vi "Edit_String_Options_list.vi"(2 "Channel Name":string, 3 "String array":string[](array[string])) -> (0 "New Selection Index":i32, 1 "String array Out":string[](array[string]))   [LabVIEW 2010]
uses:
  Controls/ok_button.ctl
panel:
  in  "Menu Strings":string[][](table)
  out "Meassage":string
  in  "OK":T1
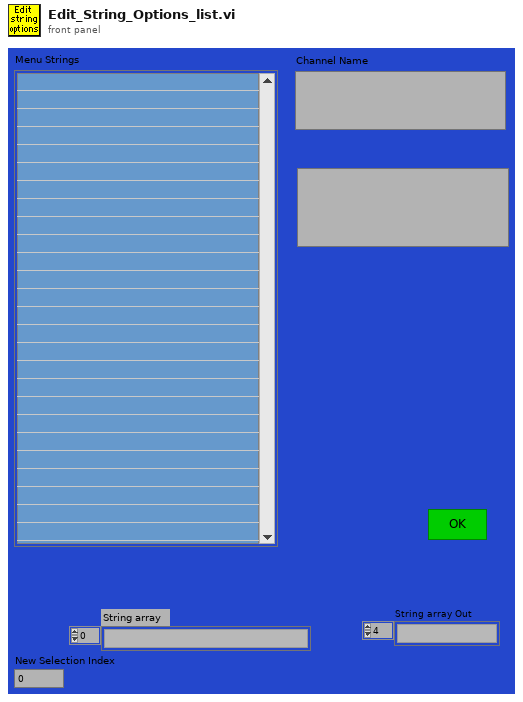
[diagram p1: front panel]
types:
  T1 = typedef "ok_button.ctl" = bool
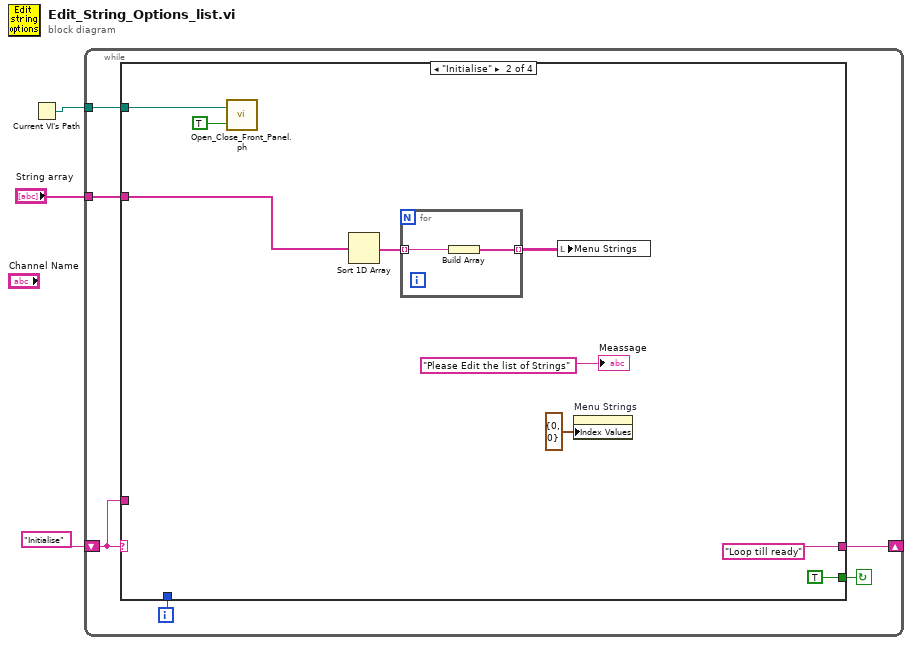
[diagram p0: block diagram]
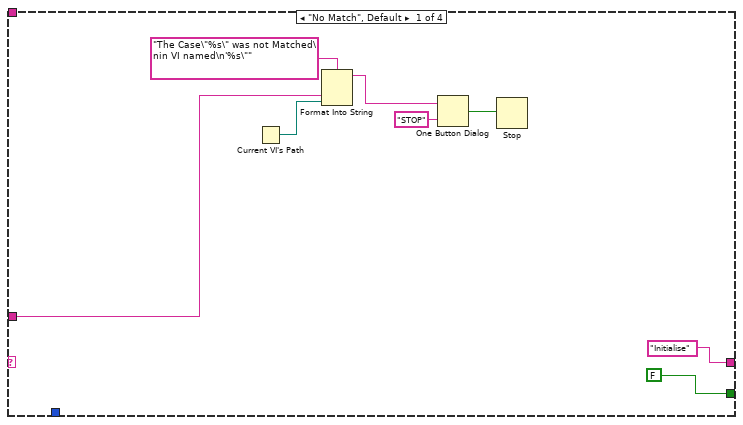
[diagram p2: hidden frame]
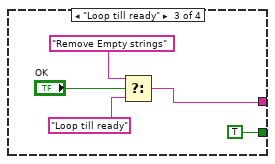
[diagram p3: hidden frame]
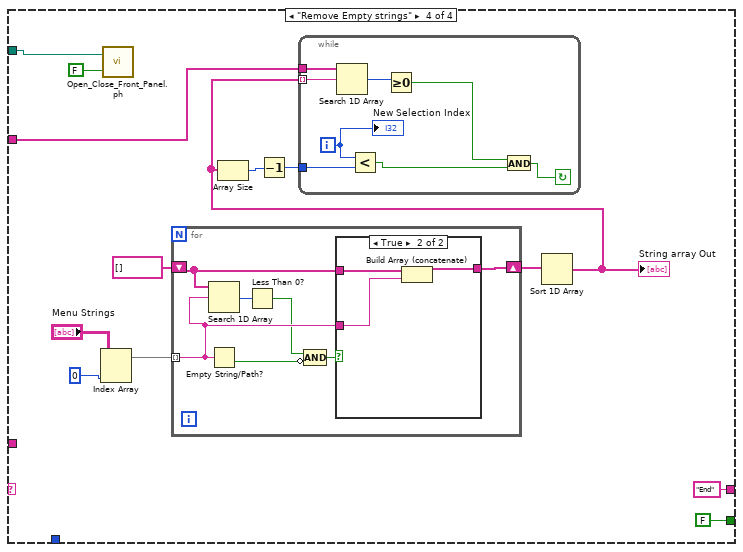
[diagram p4: hidden frame]
diagram:
  n1 = Current VI's Path() -> (path=w2:path)
  n2 = while {
    shift-left: "Initialise" -> [w7]
    shift-right: [w8] -> _
    tunnel: w2 -> [w5]
    tunnel: "String array" -> [w4]
    i -> [w6]
    stop <- w9 continue-if-true
    n3 = case shown="\"Initialise\"" w7 {
      tunnel: [FALSE TRUE TRUE FALSE] -> w9
      tunnel: ["Initialise" "Loop till ready" w30 "End"] -> w8
      tunnel: w7 -> [w12 _ _ _]
      tunnel: w6 -> [_ _ _ _]
      tunnel: w5 -> [_ w20 _ w38]
      tunnel: w4 -> [_ w18 _ w37]
      frame "No Match", Default {
        n4 = Current VI's Path() -> (path=w11:path)
        n5 = Format Into String(format string="The Case\"%s\" was not Matched\nin VI named\n'%s\"" ("Format String"), w12, w11) -> (resulting string=w15:string)  [unwired: 2 in, 1 out]
        n6 = One Button Dialog(message=w15, button name ("OK")="STOP") -> (true=w13:bool)
        n7 = Stop(stop? (T)=w13) -> ()
      }
      frame "Initialise" {
        n8 = call "Open_Close_Front_Panel.ph.vi"("Front Panel Window:Open"=TRUE, "VI path"=w20) -> ()  [unwired: 2 out]
        n9 = Sort 1D Array(array=w18) -> (sorted array=w22:string[])
        n10 = for {
          tunnel: [w28] -> w21 mode=indexing
          tunnel: w22 -> [w27] mode=indexing
          n11 = Build Array(w27) -> (w28:string[])
        }
        n12 = local write "Menu Strings"(w21) -> ()
        n13 = property on="Menu Strings" class="Tbl (strict)"("Index Values"=cluster{u32, u32} {0, 0} ("Write Attribute")) -> ()  [unwired: 2 in, 2 out]
        "Meassage" <- "Please Edit the list of Strings" ("String")
      }
      frame "Loop till ready" {
        n14 = Select(t="Remove Empty strings", s="OK", f="Loop till ready") -> (s? t:f=w30:string)
      }
      frame "Remove Empty strings" {
        n15 = Index Array(array="Menu Strings", index (col)=0 ("Index")) -> (element=w41:string[])  [unwired: 1 in]
        n16 = call "Open_Close_Front_Panel.ph.vi"("Front Panel Window:Open"=FALSE, "VI path"=w38) -> ()  [unwired: 2 out]
        n17 = for {
          shift-right: [w61] -> w40
          shift-left: string[] [] -> [w60]
          tunnel: w41 -> [w59] mode=indexing
          n18 = Search 1D Array(1D array=w60, element=w59) -> (index of element=w58:i32)  [unwired: 1 out]
          n19 = Empty String/Path?(string/path=w59) -> (empty?=w56:bool)
          n20 = Less Than 0?(x=w58) -> (x < 0?=w57:bool)
          n21 = Compound Arithmetic op=AND(w57, invert w56) -> (w55:bool)
          n22 = case shown="True" w55 {
            tunnel: w60 -> [w62 w65]
            tunnel: [w62 w64] -> w61
            tunnel: w59 -> [_ w63]
            frame False {
            }
            frame True {
              n23 = Build Array (concatenate)(w65, w63) -> (w64:string[])
            }
          }
        }
        n24 = Sort 1D Array(array=w40) -> (sorted array=w36:string[])
        "String array Out" <- w36
        n25 = Array Size(array=w36) -> (size(s)=w35:i32)
        n26 = Decrement(x=w35) -> (x-1=w34:i32)
        n27 = while {
          tunnel: w36 -> [w54] mode=indexing
          tunnel: w37 -> [w53]
          tunnel: w34 -> [w51]
          i -> [w52]
          stop <- w49 continue-if-true
          n28 = Search 1D Array(1D array=w53, element=w54) -> (index of element=w48:i32)  [unwired: 1 out]
          n29 = Less?(x=w52, y=w51) -> (x < y?=w50:bool)
          n30 = Greater Or Equal To 0?(x=w48) -> (x >= 0?=w47:bool)
          n31 = And(x=w47, y=w50) -> (x .and. y?=w49:bool)
          "New Selection Index" <- w52
        }
      }
    }
  }
